vi "SR_FFT_Biegebalken.vi"() -> ()   [LabVIEW 2020]
uses:
  <vilib>/express/express shared/transition.llb/Dynamic To Waveform Array.vi
  <vilib>/express/express arith-compare/Formula/Block/exnFormulaBlock how many pts in the wave.vi
  <vilib>/express/express shared/ex_Modify Signal Name.vi
  <vilib>/express/express shared/transition.llb/Waveform Array To Dynamic.vi
  <vilib>/express/express analysis/Spectral/Block/exnSpectralBlock spectral measurements peak poly.vi
  <vilib>/express/express analysis/Spectral/Block/exnSpectralBlock spectral measurements peak DDT.vi
  <vilib>/express/express arith-compare/Formula/XNode/ExpressFormulaBlockNode.xnode
  <vilib>/express/express analysis/Spectral/XNode/ExpressSpectralMeasurementsBlockNode.xnode
panel:
  out "Signalverlaufsgraph":dynamicdata(graph)
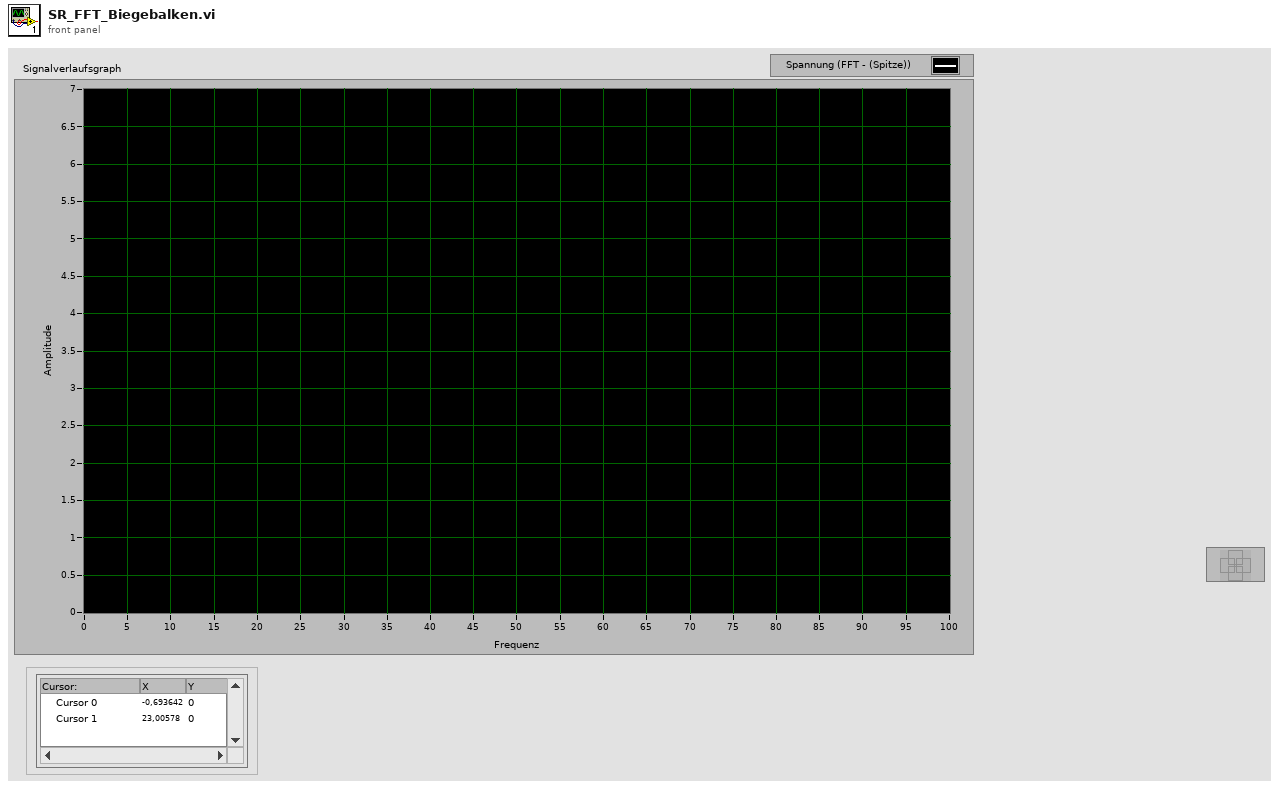
[diagram p1: front panel]
types:
  T1 = cluster{"averaging mode":u16, "weighting mode":u16, "number of averages":u32}
  T2 = cluster{"dB On (F)":bool, "unwrap phase (F)":bool, "convert to degree (F)":bool}
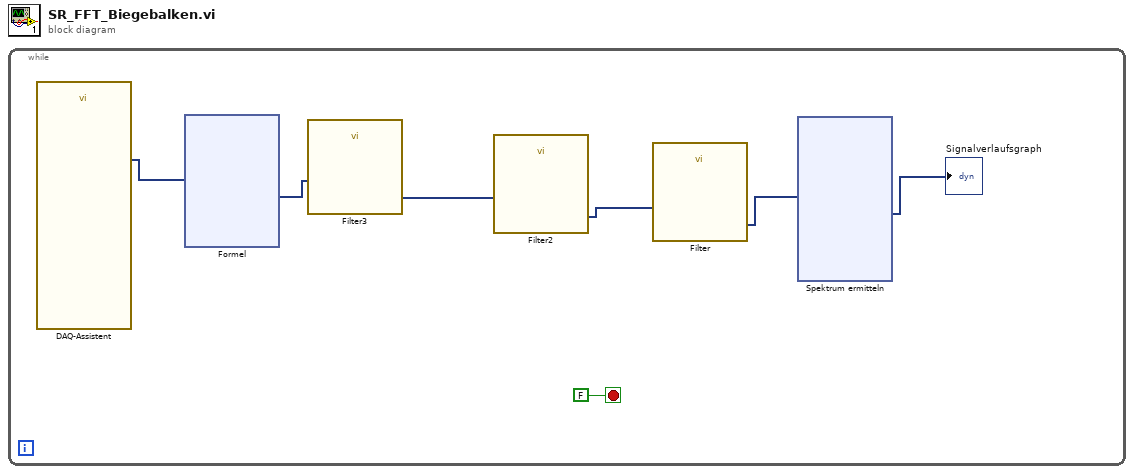
[diagram p0: block diagram]
diagram:
  n1 = while {
    stop <- FALSE stop-if-true
    n2 = call "DAQ-Assistent"() -> ("data"=w3:dynamicdata)  [unwired: 16 in, 3 out]
    n3 = xnode "Formel"("X1"=w3) -> ("Ergebnis"=w2:dynamicdata)  [unwired: 1 in, 1 out]
    n4 = call "Filter3"("Signal"=w2) -> ("Filtered Signal"=w6:dynamicdata)  [unwired: 9 in, 1 out]
    n5 = call "Filter2"("Signal"=w6) -> ("Filtered Signal"=w5:dynamicdata)  [unwired: 9 in, 1 out]
    n6 = call "Filter"("Signal"=w5) -> ("Filtered Signal"=w4:dynamicdata)  [unwired: 9 in, 1 out]
    n7 = xnode "Spektrum ermitteln"("Signale"=w4) -> ("FFT - (Spitze)"=→"Signalverlaufsgraph":dynamicdata)  [unwired: 1 in, 2 out]
  }
